vi "CameraSetScaledAttrExposure.vi"(7 "Attr Format":string="CameraAttributes::%s::Value", 8 "error in":errorcluster, 9 "Scaled":dbl, 10 "Attr String":string, 11 "IMAQdx Session in":T1) -> (0 "error out":errorcluster, 3 "IMAQdx Session":T1)   [LabVIEW 2025]
doc: "This VI updates an attribute where input unit is percentage and camera parameter may be in another unit.\n\nThis software is licensed. Open the labview\\readme\\WPI Robotics Library Open Source License.txt file for more information."
uses:
  <vilib>/userDefined/High Color/IMAQdx.ctl
  <resource>/objmgr/imaqdx.rc
  <vilib>/gmath/NI_Gmath.lvlib
panel:
  out "element":dbl
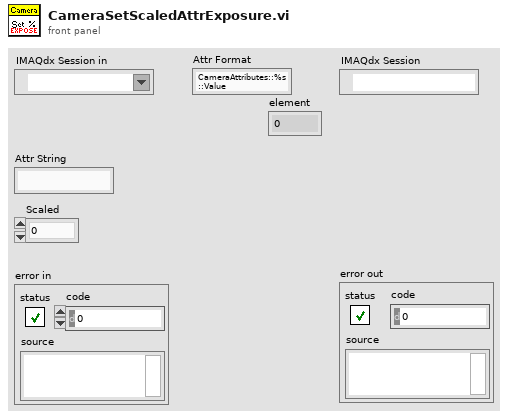
[diagram p1: front panel]
types:
  T1 = typedef "IMAQdx.ctl" = refnum<k21>
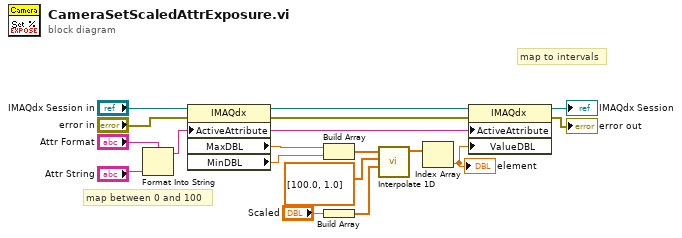
[diagram p0: block diagram]
diagram:
  # "map to intervals"
  # "map between 0 and 100"
  n1 = Format Into String(format string="Attr Format", "Attr String") -> (resulting string=w14:string)  [unwired: 2 in, 1 out]
  n2 = property class="IMAQdx"(reference="IMAQdx Session in", error in="error in", "ActiveAttribute"=w14) -> (reference out=w15:T1, error out=w12:errorcluster, "MaxDBL"=w8:dbl, "MinDBL"=w7:dbl)
  n3 = Build Array(w8, w7) -> (w6:dbl[])
  n4 = Build Array("Scaled") -> (w3:dbl[])
  n5 = call <vilib>:"Interpolate 1D.vi"("xi"=w3, "X"=dbl[] [100.0, 1.0], "Y"=w6) -> ("yi"=w2:dbl[])  [unwired: 6 in, 2 out]
  n6 = Index Array(array=w2) -> (element=w1:dbl)  [unwired: 1 in]
  "element" <- w1
  n7 = property class="IMAQdx"(reference=w15, error in=w12, "ActiveAttribute"=w14, "ValueDBL"=w1) -> (reference out=→"IMAQdx Session":T1, error out=→"error out":errorcluster)
